vi "FindCpuLoad_ALB.vi"() -> (2 "CPU2 out":dbl, 3 "CPU1 out":dbl)   [LabVIEW 2017]
uses:
  <vilib>/NI_Real-Time Target Support.lvlib
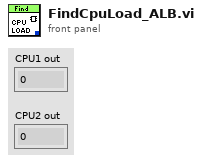
[diagram p1: front panel]
types:
  T1 = typedef "NI_Real-Time Target Support.lvlib/RT CPU Load.ctl" = cluster{"Total (%)":dbl, "Time Critical (%)":dbl, "Timed Structures (%)":dbl, "High (%)":dbl, "Above Normal (%)":dbl, "Normal (%)":dbl, "Background (%)":dbl, "Idle (%)":dbl, "ISR (%)":dbl}
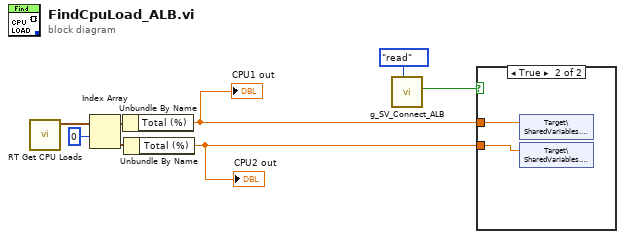
[diagram p0: block diagram]
diagram:
  n1 = call <vilib>:"RT Get CPU Loads.vi"() -> ("CPU loads"=w5:T1[])  [unwired: 10 in, 1 out]
  n2 = Index Array(array=w5, index #1=0 ("index")) -> (element #1=w6:T1, element #2=w8:T1)  [unwired: 1 in]
  n3 = Unbundle By Name(w6) -> ("Total (%)"=w4:dbl)
  "CPU1 out" <- w4
  n4 = Unbundle By Name(w8) -> ("Total (%)"=w3:dbl)
  "CPU2 out" <- w3
  n5 = call "g_SV_Connect_ALB.vi"("Action"=enum16{"read", "write"}."read") -> ("Connected"=w2:bool)  [unwired: 10 in]
  n6 = case shown="True" w2 {
    tunnel: w4 -> [_ w10]
    tunnel: w3 -> [_ w9]
    frame False {
    }
    frame True {
      n7 = shared-variable "Target\\SharedVariables.lvlib\\CPU0"(w10) -> ()  [unwired: 1 in, 1 out]
      n8 = shared-variable "Target\\SharedVariables.lvlib\\CPU1"(w9) -> ()  [unwired: 1 in, 1 out]
    }
  }
